vi "UHR-Fleezers Control (host) -Mau_stepping.vi"(0 "Tab Control":T5(tab)) -> ()   [LabVIEW 2013] (continued)
    n1508 = feedback-in #1(w2281) -> ()
    n1509 = local read "AOM X Cal (nm/MHz)"() -> (w2039:dbl)
    n1510 = To Time Stamp(1:w2086) -> (0:w2085:timestamp)
    n1511 = Split 1D Array(array=w2073, index="N El. to Ave.") -> (second subarray=w2076:dbl[])  [unwired: 1 out]
    n1512 = Split 1D Array(array=w2070, index="N El. to Ave.") -> (second subarray=w2075:dbl[])  [unwired: 1 out]
    n1513 = local read "Trap X AI1 (DMA)"() -> (w2074:T13)
    n1514 = Multiply(x=w2148, y="Trap Disp. Downsample") -> (x*y=w2087:dbl)
    "Display Period (s)" <- w2087
    n1515 = Bundle("BD 1 Frequency 1 (MHz)"=w2042, "BD 1 Frequency 2 (MHz)"=w2041) -> (w2043:T45)  [unwired: 1 out]
    n1516 = for "Trap AI" {
      tunnel: [w2695] -> w2275 mode=indexing
      tunnel: w2085 -> [w2685]
      tunnel: "Trap Disp. Downsample" -> [w2693]
      tunnel: w2166 -> [w2691] mode=indexing
      tunnel: w2148 -> [w2690]
      tunnel: w2165 -> [w2689] mode=indexing
      tunnel: w2084 -> [w2688]
      tunnel: [w2687] -> w2123 mode=indexing
      tunnel: w2087 -> [w2686]
      n1517 = Bundle By Name("Y"=w2691, "dt"=w2690) -> (w2692:waveform(dbl))  [unwired: 1 out]
      n1518 = Set Waveform Attribute(5:w2689, 6:w2688, 7:w2692) -> (3:w2687:waveform(dbl))  [unwired: 1 in, 2 out]
      n1519 = call "downsample 1D array - double.vi"("Ave N"=w2693, "Array In"=w2691) -> ("Array Out"=w2694:dbl[])  [unwired: 1 out]
      n1520 = Bundle By Name(cluster=w2687, "t0"=w2685, "Y"=w2694, "dt"=w2686) -> (w2695:waveform(dbl))
    }
    n1521 = call-poly <vilib>:"Mean.vi"("X"=w2075) -> ("mean"=w2063:dbl)  [unwired: 1 out]
    n1522 = call-poly <vilib>:"Mean.vi"("X"=w2076) -> ("mean"=w2064:dbl)  [unwired: 1 out]
    n1523 = Cluster To Array(cluster=w2043) -> (array=w2040:dbl[])
    n1524 = Reciprocal(x=w2087) -> (1/x=→"Trap Disp. Freq. (Hz)":dbl)
    n1525 = local read "Data points/scans (MCL)"() -> (w2253:dbl)
    n1526 = To Fixed-Point(number=w2063) -> (fixed-point=w2061:fxp<+/-,16,1>)  [unwired: 1 in]
    n1527 = To Fixed-Point(number=w2064) -> (fixed-point=w2062:fxp<+/-,16,1>)  [unwired: 1 in]
    n1528 = Bundle("Trap 1 Pos.", "Trap 2 Pos.") -> (w2083:cluster{string, string})  [unwired: 1 out]
    n1529 = Bundle By Name(cluster=w2074, "Set 1"=w2062, "Set 2"=w2061) -> (→"Trap X AI1 (DMA)":T13)
    n1530 = Cluster To Array(cluster=w2083) -> (array=w2080:string[])
    n1531 = for "Trap Position" {
      tunnel: w2089 -> [w2335] mode=indexing
      tunnel: "Trap Disp. Downsample" -> [w2334]
      tunnel: w2087 -> [w2332]
      tunnel: w2085 -> [w2331]
      tunnel: w2084 -> [w2329]
      tunnel: w2080 -> [w2328] mode=indexing
      tunnel: [w2327] -> w2038 mode=indexing
      tunnel: w2040 -> [w2325] mode=indexing
      tunnel: w2039 -> [w2323]
      n1532 = call "downsample 1D array - double.vi"("Ave N"=w2334, "Array In"=w2335) -> ("Array Out"=w2333:dbl[])  [unwired: 1 out]
      n1533 = Subtract(x=w2333, y=w2325) -> (x-y=w2326:dbl[])
      n1534 = Multiply(x=w2323, y=w2326) -> (x*y=w2324:dbl[])
      n1535 = Bundle By Name("Y"=w2324, "dt"=w2332, "t0"=w2331) -> (w2330:waveform(dbl))  [unwired: 1 out]
      n1536 = Set Waveform Attribute(5:w2328, 6:w2329, 7:w2330) -> (3:w2327:waveform(dbl))  [unwired: 1 in, 2 out]
    }
    "Trap Positions" <- w2038
    n1537 = Bundle("APD 1", "APD 2") -> (w2274:cluster{string, string})  [unwired: 1 out]
    n1538 = Cluster To Array(cluster=w2274) -> (array=w2271:string[])
    n1539 = for "APD" {
      tunnel: w2242 -> [w2674] mode=indexing
      tunnel: w2112 -> [w2682]
      tunnel: [w2678] -> w2119 mode=indexing
      tunnel: "APD Disp. Scale" -> [w2679]
      tunnel: w2084 -> [w2677]
      tunnel: w2271 -> [w2676] mode=indexing
      tunnel: "APD Disp. Downsample" -> [w2672]
      tunnel: [w2675] -> w2270
      tunnel: w2085 -> [w2671]
      n1540 = call "integrate 1D array interval - double.vi"("Ave N"=w2672, "Array In"=w2674) -> ("Array Out"=w2673:dbl[])  [unwired: 1 out]
      n1541 = Multiply(x=w2682, y=w2672) -> (x*y=w2675:dbl)
      n1542 = Divide(x=w2673, y=w2679) -> (x/y=w2680:dbl[])
      n1543 = Bundle By Name("t0"=w2671, "Y"=w2680, "dt"=w2675) -> (w2681:waveform(dbl))  [unwired: 1 out]
      n1544 = Set Waveform Attribute(5:w2676, 6:w2677, 7:w2681) -> (3:w2678:waveform(dbl))  [unwired: 1 in, 2 out]
    }
    "APD Display Period (s)" <- w2270
    n1545 = Reciprocal(x=w2270) -> (1/x=→"APD Display Freq. (Hz)":dbl)
    n1546 = local read "Display Period (s)"() -> (w2147:dbl)
    n1547 = Increment(x=w2253) -> (x+1=w2254:dbl)
    n1548 = Index Array(array=w2038, index=0) -> (element=w2036:waveform(dbl))
    n1549 = To Double Precision Float(number=w2163) -> (double precision float=w2162:dbl[])
    n1550 = feedback #2(w2254) -> (w2257:dbl)
    n1551 = Select(t=0, s=w2244, f=w2257) -> (s? t:f=w2250:dbl)
    n1552 = Array Size(array=w2162) -> (size(s)=w2256:i32)
    n1553 = Add(x=w2256, y=w2250) -> (x+y=w2251:dbl)
    n1554 = Unbundle By Name(w2036) -> ("Y"=w2034:dbl[])
    n1555 = feedback #3(w2163) -> (w2240:u32[])
    n1556 = Build Array (concatenate)(w2240, w2163) -> (w2237:u32[])
    n1557 = feedback #4(w2099) -> (w2118:u32[])
    n1558 = Divide(x="Bead Sep. Int. Time (s)", y=w2147) -> (x/y=w2032:dbl)
    n1559 = Build Array (concatenate)(w2118, w2099) -> (w2117:u32[])
    n1560 = Greater?(x=w2251, y=w2253) -> (0:w2252:bool)
    n1561 = feedback #5(w2034) -> (w2035:dbl[])
    n1562 = Build Array (concatenate)(w2034, w2035) -> (w2033:dbl[])
    n1563 = Select(t=w2250, s=w2252, f=w2251) -> (s? t:f=w2249:dbl)
    n1564 = feedback-in #2(w2249) -> ()
    n1565 = Array Size(array=w2237) -> (size(s)=w2234:i32)
    n1566 = Array Size(array=w2163) -> (size(s)=w2236:i32)
    n1567 = local read "MCL Scanning"() -> (w2247:bool)
    n1568 = local read "APD Integration Time (s)"() -> (w2126:dbl)
    n1569 = Build Array (concatenate)(w2119, w2275) -> (w2121:waveform(dbl)[])
    "All Signals" <- w2121
    n1570 = Split 1D Array(array=w2033, index=w2032) -> (first subarray=w2026:dbl[])  [unwired: 1 out]
    n1571 = feedback-in #5(w2026) -> ()
    n1572 = Multiply(x=w2236, y="APD Ave N") -> (x*y=w2235:dbl)
    n1573 = Greater?(x=w2234, y=w2235) -> (0:w2238:bool)
    n1574 = Not(x=w2252) -> (.not. x?=w2246:bool)
    n1575 = To Double Precision Float(number=w2099) -> (double precision float=w2098:dbl[])
    n1576 = call-poly <vilib>:"Mean.vi"("X"=w2026) -> ("mean"=w2025:dbl)  [unwired: 1 out]
    "Mean T1 Position (nm)" <- w2025
    n1577 = Subtract(x=w2026, y=w2025) -> (x-y=w2031:dbl[])
    n1578 = Square(x=w2031) -> (x^2=w2030:dbl[])
    n1579 = And(x=w2246, y=w2247) -> (x .and. y?=w2248:bool)
    n1580 = call-poly <vilib>:"Mean.vi"("X"=w2030) -> ("mean"=w2029:dbl)  [unwired: 1 out]
    n1581 = case shown="True" w2238 {
      tunnel: w2237 -> [w2455 w2462]
      tunnel: [w2455 w2460] -> w2179
      tunnel: w2235 -> [_ w2457]
      tunnel: w2234 -> [_ w2461]
      tunnel: w2117 -> [w2454 w2459]
      tunnel: [w2454 w2456] -> w2114
      frame False {
      }
      frame True {
        n1582 = Subtract(x=w2461, y=w2457) -> (x-y=w2458:dbl)
        n1583 = Array Subset(array=w2462, index=w2458, length=w2457) -> (w2460:u32[])
        n1584 = Array Subset(array=w2459, index=w2458, length=w2457) -> (w2456:u32[])
      }
    }
    n1585 = feedback-in #3(w2179) -> ()
    n1586 = feedback-in #4(w2114) -> ()
    n1587 = Or(x=w2248, y=w2244) -> (x .or. y?=w2245:bool)
    n1588 = Square Root(x=w2029) -> (sqrt(x)=w2028:dbl)
    n1589 = Equal?(x="Tab Control 6", y=T35."High Res Display") -> (x = y?=w2169:bool)
    n1590 = Multiply(x="APD Disp. Scale", y=w2119) -> (x*y=w2128:waveform(dbl)[])
    n1591 = Multiply(x="APD Disp. Downsample", y=w2126) -> (x*y=w2124:dbl)
    n1592 = Multiply(x=10.0, y=w2028) -> (x*y=→"Trap 1 Position RMS (A)":dbl)
    n1593 = Divide(x=w2128, y=w2124) -> (x/y=w2096:waveform(dbl)[])
    n1594 = Index Array(array=w2096, index=0) -> (element=w2106:waveform(dbl))
    n1595 = case "For computing FFTs for display" shown="True" "Compute FFT" {
      tunnel: w2123 -> [_ w3132]
      frame False {
      }
      frame True {
        n1596 = Build Array("FFT 1 Choice 1", "FFT 1 Choice 2", "FFT 2 Choice 1", "FFT 2 Choice 2") -> (w3125:u16[])
        n1597 = Array Size(array=w3132) -> (size(s)=w3131:i32)
        n1598 = feedback-in #6(w3125) -> ()
        n1599 = feedback #6(u16[] [100, 100, 100, 100]) -> (w3126:u16[])
        n1600 = feedback-in #7("# Spectra to Ave.") -> ()
        n1601 = feedback #7("# Spectra to Ave.") -> (w3123:dbl)
        n1602 = Not Equal?(x="# Spectra to Ave.", y=w3123) -> (x != y?=w3122:bool)
        n1603 = Not Equal?(x=w3125, y=w3126) -> (x != y?=w3124:bool)
        n1604 = feedback #8(1.0) -> (w3109:dbl)
        n1605 = Compound Arithmetic op=OR("Reset FFT", w3124, w3122) -> (w3107:bool)
        n1606 = Select(t=1.0, s=w3107, f=w3109) -> (s? t:f=w3111:dbl)
        n1607 = Greater?(x=w3111, y="# Spectra to Ave.") -> (0:w3130:bool)
        n1608 = Increment(x=w3111) -> (x+1=w3110:dbl)
        n1609 = feedback-in #8(w3110) -> ()
        n1610 = local read "DMA Update Period (s)"() -> (w3105:dbl)
        n1611 = Multiply(x="# Spectra to Ave.", y=w3105) -> (x*y=→"Ave. Time (s)":dbl)
        n1612 = Build Array(cluster{"f0":dbl, "df":dbl, "magnitude":dbl[]} {"f0"=0.0, "df"=0.0, "magnitude"=[]} ("PSD")) -> (w3114:cluster{"f0":dbl, "df":dbl, "magnitude":dbl[]}[])
        n1613 = Build Array(w3114, w3114, w3114, w3114) -> (w3116:T46)
        n1614 = feedback #9(w3116) -> (w3121:T46)
        n1615 = for {
          N: 4 -> [_]
          tunnel: w3125 -> [w3154] mode=indexing
          tunnel: w3132 -> [w3155]
          tunnel: w3131 -> [w3157]
          tunnel: w3107 -> [w3150]
          tunnel: w3130 -> [w3149]
          tunnel: "# Spectra to Ave." -> [w3148]
          tunnel: [w3147] -> w3120 mode=indexing
          tunnel: w3121 -> [w3152] mode=indexing
          tunnel: [w3151] -> w3108 mode=indexing
          tunnel: w3111 -> [w3146]
          n1616 = Less?(x=w3154, y=w3157) -> (x < y?=w3156:bool)
          n1617 = Index Array(array=w3155, index=w3154) -> (element=w3153:waveform(dbl))
          n1618 = case shown="True" w3156 {
            tunnel: w3153 -> [_ w3174]
            tunnel: w3152 -> [w3159 w3172]
            tunnel: [w3159 w3160] -> w3151
            tunnel: w3150 -> [_ w3171]
            tunnel: w3149 -> [_ w3164]
            tunnel: w3148 -> [_ w3163]
            tunnel: [cluster{"f0":dbl, "df":dbl, "magnitude":dbl[]} {"f0"=0.0, "df"=0.0, "magnitude"=[]} ("PSD") w3165] -> w3147
            tunnel: w3146 -> [_ w3162]
            frame False {
            }
            frame True {
              n1619 = call <vilib>:"Std Deviation and Variance.vi"("X"=w3174) -> ("mean"=w3175:dbl)  [unwired: 1 in, 2 out]
              n1620 = Subtract(x=w3174, y=w3175) -> (x-y=w3173:waveform(dbl))
              n1621 = xnode "Spectral Measurements"("Signals"=w3173) -> ("PSD"=w3167:cluster{"f0":dbl, "df":dbl, "magnitude":dbl[]})  [unwired: 1 in, 1 out]
              n1622 = case shown="False" w3171 {
                tunnel: w3172 -> [w3184 _]
                tunnel: [w3180 w3189] -> w3160
                tunnel: w3167 -> [w3183 w3190]
                tunnel: w3164 -> [w3182 _]
                frame False {
                  n1623 = Build Array (concatenate)(w3184, w3183) -> (w3181:cluster{"f0":dbl, "df":dbl, "magnitude":dbl[]}[])
                  n1624 = case shown="True" w3182 {
                    tunnel: w3181 -> [w3185 w3188]
                    tunnel: [w3185 w3186] -> w3180
                    frame False {
                    }
                    frame True {
                      n1625 = Delete From Array(array=w3188, index=0) -> (array with subset deleted=w3186:cluster{"f0":dbl, "df":dbl, "magnitude":dbl[]}[])  [unwired: 1 in, 1 out]
                    }
                  }
                }
                frame True {
                  n1626 = Build Array(w3190) -> (w3189:cluster{"f0":dbl, "df":dbl, "magnitude":dbl[]}[])
                }
              }
              n1627 = for {
                tunnel: w3160 -> [w3179] mode=indexing
                tunnel: [w3178] -> w3170 mode=indexing
                workers-P: _ -> [_]
                n1628 = Unbundle By Name(w3179) -> ("magnitude"=w3178:dbl[])
              }
              n1629 = Transpose 2D Array(2D array=w3170) -> (transposed array=w3169:dbl[][])
              n1630 = for {
                tunnel: w3169 -> [w3177] mode=indexing
                tunnel: [w3176] -> w3168 mode=indexing
                workers-P: _ -> [_]
                n1631 = Add Array Elements(numeric array=w3177) -> (sum=w3176:dbl)
              }
              n1632 = Select(t=w3163, s=w3164, f=w3162) -> (s? t:f=w3161:dbl)
              n1633 = Divide(x=w3168, y=w3161) -> (x/y=w3166:dbl[])
              n1634 = Bundle By Name(cluster=w3167, "magnitude"=w3166) -> (w3165:cluster{"f0":dbl, "df":dbl, "magnitude":dbl[]})
            }
          }
        }
        n1635 = case shown="True" w3107 {
          tunnel: w3108 -> [w3139 w3145]
          tunnel: [w3139 w3140] -> w3106
          frame False {
          }
          frame True {
            n1636 = Array Subset(array=w3145, index (row)=0 ("index"), length (row)=4 ("length"), index (col)=0 ("index"), length (col)=1 ("length")) -> (w3140:T46)
          }
        }
        n1637 = feedback-in #9(w3106) -> ()
        n1638 = Split 1D Array(array=w3120, index=2) -> (first subarray=→"FFT 1":cluster{"f0":dbl, "df":dbl, "magnitude":dbl[]}[], second subarray=→"FFT 2":cluster{"f0":dbl, "df":dbl, "magnitude":dbl[]}[])
      }
    }
    n1639 = Index Array(array=w2096, index=1) -> (element=w2104:waveform(dbl))
    n1640 = case "For displaying the high resolution display (no downsampling)" shown="True" w2169 {
      tunnel: w2123 -> [_ w2355]
      frame False {
      }
      frame True {
        n1641 = Index Array(array=w2355, index="High Res. Display") -> (element=w2356:waveform(dbl))
        n1642 = call <vilib>:"Std Deviation and Variance.vi"("X"=w2356) -> ("mean"=w2363:dbl, "standard deviation"=w2368:dbl)  [unwired: 1 in, 1 out]
        "Mean Intensity" <- w2363
        "Sigma" <- w2368
        n1643 = Subtract(x=w2356, y=w2363) -> (x-y=w2362:waveform(dbl))
        n1644 = Select(t=w2362, s="Subtract mean", f=w2356) -> (s? t:f=→"1 Channel":waveform(dbl))
        n1645 = Divide(x=w2368, y=w2363) -> (x/y=→"Sigma/Mean":dbl)
        n1646 = feedback #10(1) -> (w2357:i32)
        n1647 = Greater Or Equal?(x=w2357, y="Slow mean N ave.") -> (x >= y?=w2370:bool)
        n1648 = Increment(x=w2357) -> (x+1=w2372:i32)
        n1649 = Select(t=1, s=w2370, f=w2372) -> (s? t:f=w2359:i32)
        n1650 = feedback-in #10(w2359) -> ()
        n1651 = feedback #11() -> (w2360:waveform(dbl))  [unwired: 1 out]
        n1652 = case shown="Default" w2357 {
          tunnel: [w2375 w2378] -> w2361
          tunnel: w2360 -> [w2377 _]
          tunnel: w2356 -> [w2376 w2378]
          frame Default {
            n1653 = call-poly <vilib>:"Append Waveforms.vi"("waveform B"=w2376, "waveform A"=w2377) -> ("waveform out"=w2375:waveform(dbl))  [unwired: 1 in, 8 out]
          }
          frame 1 {
          }
        }
        n1654 = feedback-in #11(w2361) -> ()
        n1655 = case shown="True" w2370 {
          tunnel: w2361 -> [_ w2374]
          frame False {
          }
          frame True {
            n1656 = call-poly <vilib>:"Mean.vi"("X"=w2374) -> ("mean"=→"Slow mean":dbl)  [unwired: 1 out]
          }
        }
      }
    }
    n1657 = case "For plotting results of scanning MCL" shown="True" w2245 {
      tunnel: w2244 -> [_ w2495]
      tunnel: w2162 -> [_ w2591]
      tunnel: w2253 -> [_ _]
      tunnel: w2123 -> [_ w2565]
      tunnel: w2098 -> [_ w2496]
      tunnel: w2097 -> [_ w2469]
      frame False {
      }
      frame True {
        w2476 = u32 0 items=["Horizontal", "Vertical", "Central", "1st Diagonal", "2nd Diagonal"] ("Type of Symmetry")
        w2504 = u32 0 items=["Horizontal", "Vertical", "Central", "1st Diagonal", "2nd Diagonal"] ("Type of Symmetry")
        w2507 = u32 0 items=["Horizontal", "Vertical", "Central", "1st Diagonal", "2nd Diagonal"] ("Type of Symmetry")
        w2536 = u32 0 items=["Horizontal", "Vertical", "Central", "1st Diagonal", "2nd Diagonal"] ("Type of Symmetry")
        n1658 = Index Array(array=w2565, index=10) -> (element=w2571:waveform(dbl))
        n1659 = Index Array(array=w2565, index=11) -> (element=w2568:waveform(dbl))
        n1660 = local read "Cycles/step (MCL)"() -> (w2521:u64)
        n1661 = Index Array(array=w2565, index="Channel") -> (element=w2567:waveform(dbl))
        n1662 = Unbundle(w2469) -> ("New Image"=w2468:T3, "New Image"=w2467:T3, "New Image"=w2466:T3, "New Image"=w2465:T3)
        n1663 = Unbundle By Name(w2571) -> ("Y"=w2523:dbl[])
        n1664 = Unbundle By Name(w2568) -> ("Y"=w2525:dbl[])
        n1665 = Unbundle By Name(w2567) -> ("Y"=w2530:dbl[])
        n1666 = call "downsample 1D array - double.vi"("Ave N"=w2521, "Array In"=w2523) -> ("Array Out"=w2522:dbl[])  [unwired: 1 out]
        n1667 = call "downsample 1D array - double.vi"("Ave N"=w2521, "Array In"=w2525) -> ("Array Out"=w2524:dbl[])  [unwired: 1 out]
        n1668 = call "downsample 1D array - double.vi"("Ave N"=w2521, "Array In"=w2530) -> ("Array Out"=w2529:dbl[])  [unwired: 1 out]
        n1669 = feedback #12(w2591) -> (w2592:dbl[])
        n1670 = Build Array (concatenate)(w2592, w2591) -> (w2573:dbl[])
        n1671 = feedback #13(w2496) -> (w2498:dbl[])
        n1672 = Build Array (concatenate)(w2498, w2496) -> (w2497:dbl[])
        n1673 = local read "Scan steps (MCL)"() -> (w2478:u64)
        n1674 = Select(t=w2591, s=w2495, f=w2573) -> (s? t:f=w2577:dbl[])
        n1675 = feedback-in #12(w2577) -> ()
        n1676 = Select(t=w2496, s=w2495, f=w2497) -> (s? t:f=w2479:dbl[])
        n1677 = feedback-in #13(w2479) -> ()
        n1678 = local read "Scan lines (y)"() -> (w2464:u64)
        n1679 = local read "N APD Samp/step"() -> (w2480:dbl)
        n1680 = feedback #14(w2522) -> (w2579:dbl[])
        n1681 = Build Array (concatenate)(w2579, w2522) -> (w2570:dbl[])
        n1682 = feedback #15(w2529) -> (w2589:dbl[])
        n1683 = Build Array (concatenate)(w2589, w2529) -> (w2588:dbl[])
        n1684 = feedback #16(w2524) -> (w2581:dbl[])
        n1685 = Build Array (concatenate)(w2581, w2524) -> (w2582:dbl[])
        n1686 = Select(t=w2522, s=w2495, f=w2570) -> (s? t:f=w2526:dbl[])
        n1687 = feedback-in #14(w2526) -> ()
        n1688 = Select(t=w2529, s=w2495, f=w2588) -> (s? t:f=w2528:dbl[])
        n1689 = feedback-in #15(w2528) -> ()
        n1690 = Select(t=w2524, s=w2495, f=w2582) -> (s? t:f=w2527:dbl[])
        n1691 = feedback-in #16(w2527) -> ()
        n1692 = Multiply(x=w2478, y=u64 2) -> (x*y=w2463:u64)
        n1693 = call "integrate 1D array interval - double.vi"("Ave N"=w2480, "Array In"=w2479) -> ("Array Out"=w2491:dbl[])  [unwired: 1 out]
        n1694 = call "integrate 1D array interval - double.vi"("Ave N"=w2480, "Array In"=w2577) -> ("Array Out"=w2576:dbl[])  [unwired: 1 out]
        n1695 = Array Size(array=w2491) -> (size(s)=w2492:i32)
        n1696 = Array Size(array=w2576) -> (size(s)=w2578:i32)
        n1697 = Multiply(x=w2464, y=w2463) -> (x*y=w2494:u64)
        n1698 = Multiply(x=w2464, y=w2463) -> (x*y=w2586:u64)
        n1699 = call-poly <vilib>:"Mean.vi"("X"=w2526) -> ("mean"=w2510:dbl)  [unwired: 1 out]
        n1700 = Subtract(x=w2494, y=w2492) -> (x-y=w2485:u64)
        n1701 = call-poly <vilib>:"Mean.vi"("X"=w2528) -> ("mean"=w2515:dbl)  [unwired: 1 out]
        n1702 = call-poly <vilib>:"Mean.vi"("X"=w2527) -> ("mean"=w2513:dbl)  [unwired: 1 out]
        n1703 = call-poly <vilib>:"Mean.vi"("X"=w2491) -> ("mean"=w2482:dbl)  [unwired: 1 out]
        n1704 = Subtract(x=w2586, y=w2578) -> (x-y=w2520:u64)
        n1705 = call-poly <vilib>:"Mean.vi"("X"=w2576) -> ("mean"=w2517:dbl)  [unwired: 1 out]
        n1706 = Initialize Array(1.0 ("element"), w2485) -> (w2481:dbl[])
        n1707 = Initialize Array(1.0 ("element"), w2520) -> (w2511:dbl[])
        n1708 = Multiply(x=w2481, y=w2482) -> (x*y=w2483:dbl[])
        n1709 = Multiply(x=w2511, y=w2513) -> (x*y=w2514:dbl[])
        n1710 = Multiply(x=w2511, y=w2515) -> (x*y=w2516:dbl[])
        n1711 = Multiply(x=w2511, y=w2510) -> (x*y=w2512:dbl[])
        n1712 = Multiply(x=w2511, y=w2517) -> (x*y=w2518:dbl[])
        n1713 = Build Array (concatenate)(w2526, w2512) -> (w2580:dbl[])
        n1714 = Build Array (concatenate)(w2528, w2516) -> (w2584:dbl[])
        n1715 = Build Array (concatenate)(w2527, w2514) -> (w2583:dbl[])
        n1716 = Build Array (concatenate)(w2491, w2483) -> (w2493:dbl[])
        n1717 = Build Array (concatenate)(w2576, w2518) -> (w2585:dbl[])
        n1718 = Reshape Array(w2580, w2464, w2463) -> (w2546:dbl[][])
        n1719 = Reshape Array(w2493, w2464, w2463) -> (w2489:dbl[][])
        n1720 = Reshape Array(w2584, w2464, w2463) -> (w2538:dbl[][])
        n1721 = Reshape Array(w2583, w2464, w2463) -> (w2553:dbl[][])
        n1722 = Reshape Array(w2585, w2464, w2463) -> (w2563:dbl[][])
        n1723 = Array Subset(array=w2553, index (col)=0 ("index"), length (col)=w2478) -> (w2558:dbl[][])  [unwired: 2 in]
        n1724 = Array Subset(array=w2553, index (col)=w2478) -> (w2556:dbl[][])  [unwired: 3 in]
        n1725 = Array Subset(array=w2538, index (col)=0 ("index"), length (col)=w2478) -> (w2544:dbl[][])  [unwired: 2 in]
        n1726 = Array Subset(array=w2538, index (col)=w2478) -> (w2542:dbl[][])  [unwired: 3 in]
        n1727 = Array Subset(array=w2489, index (col)=0 ("index"), length (col)=w2478) -> (w2488:dbl[][])  [unwired: 2 in]
        n1728 = Array Subset(array=w2489, index (col)=w2478) -> (w2486:dbl[][])  [unwired: 3 in]
        n1729 = Array Subset(array=w2563, index (col)=0 ("index"), length (col)=w2478) -> (w2562:dbl[][])  [unwired: 2 in]
        n1730 = Array Subset(array=w2563, index (col)=w2478) -> (w2560:dbl[][])  [unwired: 3 in]
        n1731 = Array Subset(array=w2546, index (col)=0 ("index"), length (col)=w2478) -> (w2551:dbl[][])  [unwired: 2 in]
        n1732 = Array Subset(array=w2546, index (col)=w2478) -> (w2549:dbl[][])  [unwired: 3 in]
        n1733 = for {
          tunnel: w2558 -> [w2600] mode=indexing
          tunnel: [w2599] -> w2557 mode=indexing
          workers-P: _ -> [_]
          n1734 = Reverse 1D Array(array=w2600) -> (reversed array=w2599:dbl[])
        }
        n1735 = for {
          tunnel: w2544 -> [w2596] mode=indexing
          tunnel: [w2595] -> w2543 mode=indexing
          workers-P: _ -> [_]
          n1736 = Reverse 1D Array(array=w2596) -> (reversed array=w2595:dbl[])
        }
        n1737 = for {
          tunnel: w2488 -> [w2594] mode=indexing
          tunnel: [w2593] -> w2487 mode=indexing
          workers-P: _ -> [_]
          n1738 = Reverse 1D Array(array=w2594) -> (reversed array=w2593:dbl[])
        }
        n1739 = for {
          tunnel: w2562 -> [w2602] mode=indexing
          tunnel: [w2601] -> w2561 mode=indexing
          workers-P: _ -> [_]
          n1740 = Reverse 1D Array(array=w2602) -> (reversed array=w2601:dbl[])
        }
        n1741 = for {
          tunnel: w2551 -> [w2598] mode=indexing
          tunnel: [w2597] -> w2550 mode=indexing
          workers-P: _ -> [_]
          n1742 = Reverse 1D Array(array=w2598) -> (reversed array=w2597:dbl[])
        }
        n1743 = Index Array(array=w2563, index (row)=0) -> (element=→"Waveform Graph":dbl[])  [unwired: 1 in]
        n1744 = Add(x=w2557, y=w2556) -> (x+y=w2555:dbl[][])
        n1745 = Add(x=w2543, y=w2542) -> (x+y=w2541:dbl[][])
        n1746 = Add(x=w2487, y=w2486) -> (x+y=w2471:dbl[][])
        n1747 = Add(x=w2561, y=w2560) -> (x+y=w2535:dbl[][])
        n1748 = Add(x=w2550, y=w2549) -> (x+y=w2548:dbl[][])
        n1749 = Divide(x=w2541, y=2) -> (x/y=w2539:dbl[][])
        n1750 = Divide(x=w2555, y=2) -> (x/y=w2500:dbl[][])
        n1751 = Divide(x=w2548, y=2) -> (x/y=w2502:dbl[][])
        n1752 = To Single Precision Float(number=w2535) -> (single precision float=w2534:sgl[][])
        n1753 = Transpose 2D Array(2D array=w2539) -> (transposed array=→"Data map":dbl[][])
        n1754 = To Single Precision Float(number=w2471) -> (single precision float=w2475:sgl[][])
        n1755 = To Single Precision Float(number=w2500) -> (single precision float=w2506:sgl[][])
        n1756 = To Single Precision Float(number=w2502) -> (single precision float=w2503:sgl[][])
        n1757 = call "IMAQ ArrayToImage"("Image Pixels (Float)"=w2534, "Image"=w2468) -> ("Image Out"=w2537:T3)  [unwired: 8 in, 1 out]
        n1758 = call "IMAQ ArrayToImage"("Image Pixels (Float)"=w2475, "Image"=w2467) -> ("Image Out"=w2477:T3)  [unwired: 8 in, 1 out]
        n1759 = call "IMAQ ArrayToImage"("Image Pixels (Float)"=w2506, "Image"=w2466) -> ("Image Out"=w2508:T3)  [unwired: 8 in, 1 out]
        n1760 = call "IMAQ ArrayToImage"("Image Pixels (Float)"=w2503, "Image"=w2465) -> ("Image Out"=w2505:T3)  [unwired: 8 in, 1 out]
        n1761 = call "IMAQ Symmetry"("Type of Symmetry"=w2536, "Image Src"=w2537) -> ("Image Dst Out"=w2532:T3)  [unwired: 3 in, 1 out]
        n1762 = call "IMAQ Symmetry"("Type of Symmetry"=w2476, "Image Src"=w2477) -> ("Image Dst Out"=w2473:T3)  [unwired: 3 in, 1 out]
        n1763 = call "IMAQ Symmetry"("Type of Symmetry"=w2507, "Image Src"=w2508) -> ("Image Dst Out"=→"Detection Laser X":T3)  [unwired: 3 in, 1 out]
        n1764 = call "IMAQ Symmetry"("Type of Symmetry"=w2504, "Image Src"=w2505) -> ("Image Dst Out"=→"Detection Laser Y":T3)  [unwired: 3 in, 1 out]
        n1765 = call "IMAQ Set Simple Calibration"("Calibration Axis Info"=T36 {"Origin Pixel"={"X"=0.0, "Y"=0.0}, "Angle Relative to Horizontal (deg)"=0.0, "Axis Reference"=0}, "Grid Descriptor"=T37 {"X Step"=0.3, "Y Step"=0.3, "Unit"=enum."Undefined"}, "Image"=w2532) -> ("Calibrated Image"=→"APD 1":T3)  [unwired: 7 in, 1 out]
        n1766 = call "IMAQ Set Simple Calibration"("Calibration Axis Info"=T36 {"Origin Pixel"={"X"=0.0, "Y"=0.0}, "Angle Relative to Horizontal (deg)"=0.0, "Axis Reference"=0}, "Grid Descriptor"=T37 {"X Step"=0.3, "Y Step"=0.3, "Unit"=enum."Undefined"}, "Image"=w2473) -> ("Calibrated Image"=→"APD 2":T3)  [unwired: 7 in, 1 out]
      }
    }
    n1767 = Subtract(x=w2104, y="APD 2 Offset") -> (x-y=w2101:waveform(dbl))
    n1768 = Subtract(x=w2106, y="APD 1 Offset") -> (x-y=w2102:waveform(dbl))
    n1769 = Index Array(array=w2121, index=3) -> (element=w2189:waveform(dbl))
    n1770 = Index Array(array=w2121, index=6) -> (element=w2186:waveform(dbl))
    n1771 = Build Array(w2102, w2101) -> (→"APD Chart":waveform(dbl)[])
    n1772 = Array Size(array=w2179) -> (size(s)=w2233:i32)
    n1773 = call <vilib>:"Std Deviation and Variance.vi"("X"=w2114) -> ("standard deviation"=w2113:dbl)  [unwired: 1 in, 2 out]
    n1774 = Add Array Elements(numeric array=w2114) -> (sum=w2116:u32)
    n1775 = Add Array Elements(numeric array=w2179) -> (sum=w2243:u32)
    n1776 = call <vilib>:"Std Deviation and Variance.vi"("X"=w2179) -> ("standard deviation"=w2178:dbl)  [unwired: 1 in, 2 out]
    n1777 = Divide(x="T1 offset_x (mV)", y=1000.0) -> (x/y=w2190:dbl)
    n1778 = Divide(x=w2113, y=w2112) -> (x/y=w2109:dbl)
    "Rate sigma (Hz) 2" <- w2109
    n1779 = Multiply(x=w2112, y=w2233) -> (x*y=w2115:dbl)
    "Int. Time (s)" <- w2115
    n1780 = Divide(x=w2116, y=w2115) -> (x/y=w2110:dbl)
    "APD 2 Rate (Hz)" <- w2110
    n1781 = Divide(x=w2243, y=w2115) -> (x/y=w2176:dbl)
    "APD 1 Rate (Hz)" <- w2176
    n1782 = Divide(x=w2178, y=w2112) -> (x/y=w2177:dbl)
    "Rate sigma (Hz)" <- w2177
    n1783 = Divide(x=w2109, y=w2110) -> (x/y=→"Sigma/Mean 2":dbl)
    n1784 = Divide(x=w2177, y=w2176) -> (x/y=→"Sigma/Mean":dbl)
    n1785 = Divide(x="T2 offset_x (mV)", y=1000.0) -> (x/y=w2188:dbl)
    n1786 = case shown="1" "Calibration" {
      tunnel: "T1 alpha_x (nm/V)" -> [_ w2431 w2452]
      tunnel: "T1 kappa_x (pN/nm)" -> [_ _ w2442]
      tunnel: "T2 alpha_x (nm/V)" -> [_ w2430 w2450]
      tunnel: "T2 kappa_x (pN/nm)" -> [_ _ w2443]
      tunnel: w2189 -> [w2413 w2428 w2448]
      tunnel: w2186 -> [w2412 w2426 w2446]
      tunnel: [w2413 w2425 w2445] -> w2219
      tunnel: [w2412 w2424 w2444] -> w2218
      tunnel: ["T1 X (V)" ("Label.Text") "T1 X (nm)" ("Label.Text") "T1 X (pN)" ("Label.Text")] -> w2207
      tunnel: ["T2 X (V)" ("Label.Text") "T2 X (nm)" ("Label.Text") "T2 X (pN)" ("Label.Text")] -> w2206
      tunnel: ["Position (V)" ("Label.Text") "Position (nm)" ("Label.Text") "Force (pN)" ("Label.Text")] -> w2208
      tunnel: w2188 -> [_ w2416 w2435]
      tunnel: w2190 -> [_ w2419 w2437]
      tunnel: ["Mean (V)" ("Label.Text") "Mean (nm)" ("Label.Text") "Mean (pN)" ("Label.Text")] -> w2203
      tunnel: ["Difference (V)" ("Label.Text") "Difference (nm)" ("Label.Text") "Difference (pN)" ("Label.Text")] -> w2129
      frame 0, Default {
      }
      frame 1 {
        # "position"
        n1787 = Unbundle By Name(w2428) -> ("Y"=w2432:dbl[])
        n1788 = Unbundle By Name(w2426) -> ("Y"=w2417:dbl[])
        n1789 = Subtract(x=w2432, y=w2419) -> (x-y=w2420:dbl[])
        n1790 = Subtract(x=w2417, y=w2416) -> (x-y=w2418:dbl[])
        n1791 = Multiply(x=w2418, y=w2430) -> (x*y=w2427:dbl[])
        n1792 = Multiply(x=w2431, y=w2420) -> (x*y=w2429:dbl[])
        n1793 = Bundle By Name(cluster=w2426, "Y"=w2427) -> (w2424:waveform(dbl))
        n1794 = Bundle By Name(cluster=w2428, "Y"=w2429) -> (w2425:waveform(dbl))
      }
      frame 2 {
        # "force"
        n1795 = Unbundle By Name(w2448) -> ("Y"=w2453:dbl[])
        n1796 = Unbundle By Name(w2446) -> ("Y"=w2451:dbl[])
        n1797 = Subtract(x=w2451, y=w2435) -> (x-y=w2436:dbl[])
        n1798 = Subtract(x=w2453, y=w2437) -> (x-y=w2438:dbl[])
        n1799 = Compound Arithmetic op=MULTIPLY(w2436, w2450, w2443) -> (w2447:dbl[])
        n1800 = Compound Arithmetic op=MULTIPLY(w2442, w2452, w2438) -> (w2449:dbl[])
        n1801 = Bundle By Name(cluster=w2446, "Y"=w2447) -> (w2444:waveform(dbl))
        n1802 = Bundle By Name(cluster=w2448, "Y"=w2449) -> (w2445:waveform(dbl))
      }
    }
    n1803 = feedback-in #17("Calibration") -> ()
    n1804 = feedback #17(u16 1 ("Calibration")) -> (w2210:u16)
    n1805 = local read "Trap 2 Bead Size (nm)"() -> (w2008:dbl)
    n1806 = local read "Trap 1 Bead Size (nm)"() -> (w2007:dbl)
    n1807 = local read "AOM X Cal (nm/MHz)"() -> (w2005:dbl)
    n1808 = local read "Trap Delta (MHz)"() -> (w2004:dbl)
    n1809 = Not Equal?(x=w2210, y="Calibration") -> (x != y?=w2167:bool)
    n1810 = Multiply(x=w2005, y=w2004) -> (x*y=w2009:dbl)
    n1811 = Add(x=w2008, y=w2007) -> (x+y=w2011:dbl)
    n1812 = Unbundle By Name(w2189) -> ("Y"=w2192:dbl[])
    n1813 = Unbundle By Name(w2186) -> ("Y"=w2195:dbl[])
    n1814 = Divide(x=w2011, y=2.0) -> (x/y=w2006:dbl)
    n1815 = Subtract(x=w2192, y=w2190) -> (x-y=w2193:dbl[])
    n1816 = Subtract(x=w2195, y=w2188) -> (x-y=w2194:dbl[])
    n1817 = disable-structure shown="Enabled" {
      disable-tunnel: [-1.0 ("y") 1.0] -> w2196
      frame Disabled {
      }
      frame Enabled {
      }
    }
    n1818 = Multiply(x=w2194, y="T2 alpha_x (nm/V)") -> (x*y=w2185:dbl[])
    n1819 = Multiply(x="T1 alpha_x (nm/V)", y=w2193) -> (x*y=w2184:dbl[])
    n1820 = Multiply(x=w2218, y=w2196) -> (x*y=w2197:waveform(dbl))
    n1821 = case shown="False" "Read Lateness and Rel Phase" {
      tunnel: w2021 -> [w2379 w2401]
      tunnel: w2020 -> [w2380 w2400]
      tunnel: [w2379 w2399] -> w2182
      tunnel: [w2380 w2398] -> w2181
      frame False {
      }
      frame True {
        n1822 = xnode "Read/Write Control"("FPGA VI Reference In"=w2401, "error in"=w2400) -> ("FPGA VI Reference Out"=w2399:T19, "error out"=w2398:errorcluster, "GI Relative phase"=→"GI relative phase":i16, "Relative phase"=→"Relative phase (AI1)":i16, "AI Late Counter"=→"Late Counter (AI1)":u16, "GI Late Counter"=→"GI Late Counter":u16, "MCL Late Counter"=→"MCL Late Counter":u16, "MCL Relative Phase"=→"Relative Phase (MCL)":i16, "APD Acq Relative Phase"=→"APD Acq Relative Phase":i16, "APD 1 Gate Relative Phase"=→"APD 1 Gate Relative Phase":i16, "APD 2 Gate Relative Phase"=→"APD 2 Gate Relative Phase":i16, "APD Acq Late Counter"=→"APD Acq Late Counter":u16, "APD 1 Gate Late Counter"=→"APD 1 Gate Late Counter":u16, "APD 2 Gate Late Counter"=→"APD 2 Gate Late Counter":u16, "Green FB Relative Phase"=→"Relative phase (Green FB)":i16, "GI Relative phase 2"=→"GI relative phase 2":i16, "GI Late Counter 2"=→"GI Late Counter 2":u16, "Trap Pos FIFO Timeout"=→"Trap Pos FIFO Timeout":u16, "Trap AI FIFO Timeout"=→"Trap AI FIFO Timeout":u16)
      }
    }
    n1823 = Subtract(x=w2185, y=w2184) -> (x-y=w2003:dbl[])
    n1824 = call-poly <vilib>:"Mean.vi"("X"=w2003) -> ("mean"=w2010:dbl)  [unwired: 1 out]
    n1825 = Add(x=w2009, y=w2010) -> (x+y=w2013:dbl)
    n1826 = Subtract(x=w2013, y=w2006) -> (x-y=→"Tether Extension (nm, calculated)":dbl)
    n1827 = Unbundle By Name(w2218) -> ("Y"=w2154:dbl[])
    n1828 = Unbundle By Name(w2219) -> ("Y"=w2155:dbl[])
    n1829 = Build Array(w2219, w2197) -> (→"Force":waveform(dbl)[])
    n1830 = Subtract(x=w2003, y="Offset (nm)") -> (x-y=w2152:dbl[])
    n1831 = call-poly <vilib>:"Mean.vi"("X"=w2154) -> ("mean"=w2133:dbl)  [unwired: 1 out]
    "T2 X" <- w2133
    n1832 = Absolute Value(x=w2155) -> (abs(x)=w2156:dbl[])
    n1833 = Absolute Value(x=w2154) -> (abs(x)=w2157:dbl[])
    n1834 = call-poly <vilib>:"Mean.vi"("X"=w2155) -> ("mean"=w2134:dbl)  [unwired: 1 out]
    "T1 X" <- w2134
    n1835 = Add(x=w2156, y=w2157) -> (x+y=w2158:dbl[])
    n1836 = Bundle By Name(cluster=w2189, "Y"=w2152) -> (w2120:waveform(dbl))
    "Bead Separation" <- w2120
    n1837 = Divide(x=w2158, y=2.0) -> (x/y=→"Vec Mean of T1 T2":dbl[])
    n1838 = case shown="True" w2167 {
      tunnel: w2208 -> [_ w2406]
      tunnel: w2207 -> [_ w2405]
      tunnel: w2206 -> [_ w2404]
      tunnel: w2203 -> [_ w2403]
      tunnel: w2129 -> [_ w2402]
      frame False {
      }
      frame True {
        n1839 = property on="Force" class="WFChart (strict)"("YScale.NameLbl.Text"=w2406) -> ()  [unwired: 2 in, 2 out]
        n1840 = property on="T2 X" class="DigNum (strict)"("Caption.Text"=w2404) -> ()  [unwired: 2 in, 2 out]
        n1841 = property on="T1 X" class="DigNum (strict)"("Caption.Text"=w2405) -> ()  [unwired: 2 in, 2 out]
        n1842 = property on="Mean" class="DigNum (strict)"("Caption.Text"=w2403) -> ()  [unwired: 2 in, 2 out]
        n1843 = property on="Difference" class="DigNum (strict)"("Caption.Text"=w2402) -> ()  [unwired: 2 in, 2 out]
      }
    }
    n1844 = local read "Tether"() -> (w2161:bool)
    n1845 = Absolute Value(x=w2134) -> (abs(x)=w2131:dbl)
    n1846 = Absolute Value(x=w2133) -> (abs(x)=w2130:dbl)
    n1847 = Add(x=w2131, y=w2130) -> (x+y=w2205:dbl)
    n1848 = Subtract(x=w2131, y=w2130) -> (x-y=→"Difference":dbl)
    n1849 = feedback #18(w2152) -> (w2151:dbl[])
    n1850 = Divide(x=w2205, y=2.0) -> (x/y=w2160:dbl)
    "Mean" <- w2160
    n1851 = case shown="True" w2161 {
      tunnel: w2160 -> [_ w2338]
      frame False {
      }
      frame True {
        n1852 = Greater?(x="Lost Tether Alarm Threshold (pN)", y=w2338) -> (0:w2336:bool)
        n1853 = case shown="True" w2336 {
          frame False {
          }
          frame True {
            n1854 = flat-sequence {
              frame #0 {
                # "stop only if saving"
                n1855 = local read "Saving..."() -> (w2351:bool)
                n1856 = And(x=w2351, y="TA Cancel Save?") -> (x .and. y?=w2350:bool)
                n1857 = local write "Stop Saving"(w2350) -> ()
              }
              frame #1 {
                n1858 = case shown="True" "TA Green Off?" {
                  frame False {
                  }
                  frame True {
                    w2354 = FALSE ("Fl. Triggered...")
                    n1859 = local write "Fl. Triggered..."(w2354) -> ()
                    n1860 = property on="Green Laser ON/Interlacing" class="Bool (strict)"("Val(Sgnl)"=w2354) -> ()  [unwired: 2 in, 2 out]
                  }
                }
              }
            }
            n1861 = local read "Time tether formed"() -> (w2345:timestamp)
            n1862 = Get Date/Time In Seconds() -> (seconds since 1Jan1904=w2346:timestamp)
            n1863 = Subtract(x=w2346, y=w2345) -> (x-y=w2344:dbl)
            n1864 = Number To Decimal String(number=w2344) -> (decimal integer string=w2341:string)  [unwired: 1 out]
            n1865 = local read "Messages"() -> (w2348:string)
            n1866 = call <vilib>:"Beep.vi"() -> ()  [unwired: 3 in, 9 out]
            n1867 = Concatenate Strings("Lost tether (" ("Message to add"), w2341, " s)." ("string")) -> (w2343:string)
            n1868 = local write "Tether"(FALSE ("Tether")) -> ()
            n1869 = call "Update messages.vi"("Message to add"=w2343, "Old message string"=w2348) -> ("New message string"=w2347:string)
            n1870 = local write "Messages"(w2347) -> ()
            n1871 = property on="Trap Pos. FB ON" class="Bool (strict)"("Val(Sgnl)"=FALSE ("Value (Signaling)")) -> ()  [unwired: 2 in, 2 out]
          }
        }
      }
    }
    n1872 = Build Array (concatenate)(w2152, w2151) -> (w2150:dbl[])
    n1873 = Split 1D Array(array=w2150, index=w2032) -> (first subarray=w2146:dbl[])  [unwired: 1 out]
    n1874 = feedback-in #18(w2146) -> ()
    n1875 = call-poly <vilib>:"Mean.vi"("X"=w2146) -> ("mean"=w2145:dbl)  [unwired: 1 out]
    "Bead Mean (nm)" <- w2145
    n1876 = Subtract(x=w2146, y=w2145) -> (x-y=w2144:dbl[])
    n1877 = Square(x=w2144) -> (x^2=w2143:dbl[])
    n1878 = call-poly <vilib>:"Mean.vi"("X"=w2143) -> ("mean"=w2142:dbl)  [unwired: 1 out]
    n1879 = Square Root(x=w2142) -> (sqrt(x)=w2141:dbl)
    n1880 = Multiply(x=10.0, y=w2141) -> (x*y=→"RMS (Ang)":dbl)
    n1881 = xnode "Read/Write Control"("FPGA VI Reference In"=w2182, "error in"=w2181) -> ("FPGA VI Reference Out"=w2299:T19, "error out"=w2293:errorcluster, "AI4 Y Sum Set 1"=w2289:i16, "AI4 Y Sum Set 2"=w2288:i16, "AI1 X Set 1"=w2066:fxp<+/-,16,1>, "AI1 X Set 2"=w2065:fxp<+/-,16,1>, "Trap Pos FB Int Signal"=→"Trap Pos FB Int Signal":fxp<+/-,24,9>, "Trap Pos FB Int-Norm Signal"=→"Trap Pos FB Int-Norm Signal":fxp<+/-,16,1>, "Trap Pos FB Action"=w2059:i64, "Scanning"=→"AOD Scanning":bool, "Scan I"=→"AOD Scan I":u64, "Scanning MCL"=w2291:bool, "Scan I (MCL)"=→"MCL Scan I":u64, "Green FB Signals"=w2228:T47)  [unwired: 1 out]
    "MCL Scanning" <- w2291
    "Trap Pos FB Action" <- w2059
    n1882 = local read "AI2 (V)"() -> (w2290:cluster{"Set 1":dbl, "Set 2":dbl})
    n1883 = Bundle By Name(cluster=w2290, "Set 1"=w2289, "Set 2"=w2288) -> (w2286:cluster{"Set 1":dbl, "Set 2":dbl})
    n1884 = Divide(x=w2059, y=327.67) -> (x/y=→"Action (%)":dbl)
    n1885 = local read "Trap X (AI1)"() -> (w2079:T1)
    n1886 = Divide(x=w2286, y=3276.7) -> (x/y=w2285:cluster{"Set 1":dbl, "Set 2":dbl})
    n1887 = local write "AI2 (V)"(w2285) -> ()
    n1888 = Bundle(cluster=w2079, "Trap 1"=w2066, "Trap 2"=w2065) -> (→"Trap X (AI1)":T1)
    n1889 = Divide(x=w2228, y=3276.7) -> (x/y=w2224:T48)
    n1890 = Unbundle By Name(w2224) -> ("Green FB Ch 0"=w2227:dbl, "Green FB Ch 1"=w2226:dbl, "Green FB Ch 2"=w2225:dbl)
    n1891 = Divide(x=w2227, y=w2225) -> (x/y=w2223:dbl)
    n1892 = Divide(x=w2226, y=w2225) -> (x/y=w2222:dbl)
    n1893 = flat-sequence "To save data" {
      tunnel: [w3228] -> w2310
      tunnel: [w3229] -> w2309
      tunnel: w2259 -> [w3222]
      tunnel: w2148 -> [w3226]
      tunnel: ["Save Calibration"] -> w2282
      tunnel: w2279 -> [w3225]
      tunnel: [w3218] -> w2278
      tunnel: [w3215] -> w2277
      tunnel: [w3212] -> w2276
      tunnel: w2258 -> [w3214]
      tunnel: w2165 -> [w3208]
      tunnel: [w3208] -> w2164
      tunnel: ["Start Saving"] -> w2122
      tunnel: [w3202] -> w2048
      tunnel: [w3201] -> w2047
      tunnel: w2310 -> [w3463]
      tunnel: w2309 -> [w3462]
      tunnel: w2049 -> [w3461]
      tunnel: w2282 -> [w3460]
      tunnel: w2278 -> [w3458]
      tunnel: w2277 -> [w3457]
      tunnel: w2276 -> [w3456]
      tunnel: w2135 -> [w3455]
      tunnel: w2174 -> [w3454]
      tunnel: w2164 -> [w3453]
      tunnel: w2122 -> [w3452]
      tunnel: w2120 -> [w3451]
      tunnel: w2096 -> [w3450]
      tunnel: w2048 -> [w3449]
      tunnel: w2047 -> [w3448]
      tunnel: w2046 -> [w3447]
      frame #0 {
        n1894 = Or(x="Save N Sets", y="Start Saving") -> (x .or. y?=w3209:bool)
        n1895 = To Double Precision Float(number=w3225) -> (double precision float=w3219:dbl)
        n1896 = Build Array(w3209, "Save Calibration", w3222, w3214) -> (w3224:bool[])
        n1897 = Compound Arithmetic op=OR("Save Calibration", w3222, w3209, w3214) -> (w3227:bool)
        n1898 = Boolean Array To Number(Boolean array=w3224) -> (number=w3221:u32)
        n1899 = feedback #19(FALSE ("Save APD Data\nwith Trap Data")) -> (w3203:bool)
        n1900 = feedback #20(refnum<k0> refnum) -> (w3230:refnum<file>)
        n1901 = feedback #21(refnum<k0> refnum) -> (w3205:refnum<file>)
        n1902 = feedback #22(FALSE ("Save APD Data\nwith Trap Data")) -> (w3213:bool)
        n1903 = feedback #23(refnum<k0> refnum) -> (w3216:refnum<file>)
        n1904 = feedback #24(0) -> (w3232:i32)
        n1905 = feedback #25() -> (w3220:u32)  [unwired: 1 out]
        n1906 = case shown="True" w3227 {
          tunnel: [w3239 1] -> w3228
          tunnel: w3232 -> [w3241 _]
          tunnel: [w3240 w3259] -> w3229
          tunnel: w3230 -> [w3240 _]
          tunnel: w3226 -> [_ w3279]
          tunnel: w3219 -> [_ w3277]
          tunnel: w3221 -> [_ w3280]
          tunnel: [w3238 w3258] -> w3218
          tunnel: w3220 -> [w3238 _]
          tunnel: [w3237 w3256] -> w3215
          tunnel: w3216 -> [w3237 _]
          tunnel: [w3236 w3255] -> w3212
          tunnel: w3213 -> [w3236 _]
          tunnel: "Start Saving" -> [_ w3253]
          tunnel: w3208 -> [_ w3252]
          tunnel: [w3235 w3243] -> w3201
          tunnel: w3205 -> [w3235 _]
          tunnel: [w3234 w3242] -> w3202
          tunnel: w3203 -> [w3234 _]
          frame False {
            n1907 = Increment(x=w3241) -> (x+1=w3239:i32)
          }
          frame True {
            w3249 = FALSE ("Start Saving")
            w3254 = 9.0  # File Version
            w3262 = FALSE ("prepend array or string size? (T)")
            w3260 = T29."big-endian, network order" ("byte order (0:big-endian, network order)")
            # "write file headers"
            n1908 = local read "BD 1 Frequency 1 (MHz)"() -> (w3276:dbl)
            n1909 = local read "BD 2 Frequency 1 (MHz)"() -> (w3275:dbl)
            n1910 = local read "BD 1 Frequency 2 (MHz)"() -> (w3274:dbl)
            n1911 = local read "BD 2 Frequency 2 (MHz)"() -> (w3273:dbl)
            n1912 = local read "BD 1 Frequency 3 (MHz)"() -> (w3272:dbl)
            n1913 = local read "BD 2 Frequency 3 (MHz)"() -> (w3271:dbl)
            n1914 = Array Size(array=w3252) -> (size(s)=w3251:i32)
            n1915 = To Double Precision Float(number=w3251) -> (double precision float=w3250:dbl)
            n1916 = local write "Save Calibration"(w3249) -> ()
            n1917 = local write "Start Saving"(w3249) -> ()
            n1918 = Build Array("Save APD Data\nwith Trap Data", "Save Trap Pos. Data") -> (w3246:bool[])
            n1919 = Boolean Array To Number(Boolean array=w3246) -> (number=w3245:u32)
            n1920 = Build Array(w3276, w3275, w3274, w3273, w3272, w3271) -> (w3270:dbl[])
            n1921 = case shown="4" w3280 {
              tunnel: w3279 -> [w3351 w3371 w3387 w3425]
              tunnel: w3250 -> [w3356 w3378 w3407 w3444]
              tunnel: w3277 -> [w3355 w3377 w3406 w3443]
              tunnel: [w3352 w3373 w3398 w3435] -> w3268
              tunnel: [w3343 "Cal sets to save" w3388 w3426] -> w3258
              tunnel: w3270 -> [w3353 w3374 w3400 w3437]
              tunnel: "Save APD Data\nwith Trap Data" -> [w3350 _ w3384 w3423]
              tunnel: [w3350 w3365 w3384 w3423] -> w3255
              tunnel: w3254 -> [w3346 w3366 w3382 w3421]
              tunnel: w3253 -> [w3345 _ _ _]
              tunnel: [w3336 w3365 w3381 w3411] -> w3242
              tunnel: "Save Trap Pos. Data" -> [w3336 _ w3381 w3411]
              tunnel: w3245 -> [w3335 _ w3380 w3410]
              frame 1, Default {
                # "timeseries"
                n1922 = case shown="True" "Profile" {
                  tunnel: [w3359 w3362] -> w3340
                  tunnel: [w3359 w3361] -> w3339
                  tunnel: [w3359 w3360] -> w3338
                  tunnel: [w3359 w3364] -> w3337
                  frame False {
                    w3359 = 0.0 ("f")
                  }
                  frame True {
                    n1923 = local read "Current Position"() -> (w3363:dbl[])
                    n1924 = local read "Y change (mm)"() -> (w3364:dbl)
                    n1925 = call "subVI_explode3array.vi"("Array"=w3363) -> ("x"=w3362:dbl, "y"=w3361:dbl, "z"=w3360:dbl)  [unwired: 12 in]
                  }
                }
                n1926 = local read "Save ave N"() -> (w3358:dbl)
                n1927 = Multiply(x=w3358, y=w3351) -> (x*y=w3357:dbl)
                n1928 = To Double Precision Float(number=w3335) -> (double precision float=w3349:dbl)
                n1929 = Build Array(w3346, w3351, w3357, w3356, w3355, 0.0 ("f")) -> (w3354:dbl[])
                n1930 = Build Array(w3349, w3340, w3339, w3338, w3337) -> (w3347:dbl[])
                n1931 = Select(t=u32 4000000000, s=w3345, f="N sets to save") -> (s? t:f=w3343:u32)
                n1932 = Build Array (concatenate)(w3354, w3353, w3347) -> (w3352:dbl[])
              }
              frame 2 {
                w3368 = 0.0 ("f")
                w3365 = FALSE ("Save APD Data\nwith Trap Data")
                # "calibration"
                n1933 = Boolean To (0,1)(Boolean=w3365) -> (0, 1=w3370:i16)
                n1934 = To Double Precision Float(number=w3370) -> (double precision float=w3369:dbl)
                n1935 = Build Array(w3369, w3368, w3368, w3368, w3368) -> (w3367:dbl[])
                n1936 = Build Array(w3366, w3371, w3371, w3378, w3377, 1.0 ("t")) -> (w3375:dbl[])
                n1937 = Build Array (concatenate)(w3375, w3374, w3367) -> (w3373:dbl[])
                "Calibrating Trap..." <- TRUE ("Calibrating...")
              }
              frame 4 {
                w3385 = 0.0 ("f")
                # "write file header for a trap \nraster scan"
                # "scan dir (x/y = 0/1)"
                # "cycles/step"
                # "n scans (f/b)"
                # "steps"
                # "freq. range"
                # "AOD raster scan"
                n1938 = local read "Number of F/B Scans (AOD)"() -> (w3392:u16)
                n1939 = local read "Cycles/step (AOD)"() -> (w3394:u64)
                n1940 = local read "Scan Range (MHz)"() -> (w3397:dbl)
                n1941 = local read "Scan steps (AOD)"() -> (w3396:u64)
                n1942 = local read "Scan BD"() -> (w3404:bool)
                n1943 = local read "Save ave N"() -> (w3409:dbl)
                n1944 = Boolean To (0,1)(Boolean=w3404) -> (0, 1=w3403:i16)
                n1945 = To Double Precision Float(number=w3392) -> (double precision float=w3391:dbl)
                n1946 = To Double Precision Float(number=w3396) -> (double precision float=w3395:dbl)
                n1947 = To Double Precision Float(number=w3394) -> (double precision float=w3393:dbl)
                n1948 = To Double Precision Float(number=w3403) -> (double precision float=w3402:dbl)
                n1949 = Multiply(x=w3409, y=w3387) -> (x*y=w3408:dbl)
                n1950 = To Double Precision Float(number=w3380) -> (double precision float=w3386:dbl)
                n1951 = Build Array(w3386, w3385, w3385, w3385, w3385) -> (w3383:dbl[])
                n1952 = local read "N sets should be saved"() -> (w3389:dbl)
                n1953 = Build Array(w3402, w3397, w3395, w3393, w3391) -> (w3399:dbl[])
                n1954 = Build Array(w3382, w3387, w3408, w3407, w3406, 2.0 ("t")) -> (w3401:dbl[])
                n1955 = Round Toward +Infinity(x=w3389) -> (ceil(x): smallest int >= x=w3390:dbl)
                n1956 = Build Array (concatenate)(w3401, w3400, w3383, w3399) -> (w3398:dbl[])
                n1957 = To Unsigned Long Integer(number=w3390) -> (unsigned 32bit integer=w3388:u32)
              }
              frame 8 {
                w3418 = 0.0 ("f")
                # "MCL raster scan"
                n1958 = local read "Number of scans (MCL)"() -> (w3413:u64)
                n1959 = local read "Scan lines (y)"() -> (w3412:u64)
                n1960 = local read "2D or 1D Scan"() -> (w3415:bool)
                n1961 = local read "Scan Range (V)\n(of steps)"() -> (w3434:dbl)
                n1962 = local read "Fast Scan Dir"() -> (w3441:bool)
                n1963 = local read "Cycles/step (MCL)"() -> (w3431:u64)
                n1964 = local read "Scan steps (MCL)"() -> (w3433:u64)
                n1965 = Select(t=w3412, s=w3415, f=w3413) -> (s? t:f=w3414:u64)
                n1966 = Boolean To (0,1)(Boolean=w3415) -> (0, 1=w3417:i16)
                n1967 = local read "Save ave N"() -> (w3446:dbl)
                n1968 = local read "Initial X"() -> (w3420:dbl)
                n1969 = local read "Initial Y"() -> (w3419:dbl)
                n1970 = To Double Precision Float(number=w3417) -> (double precision float=w3416:dbl)
                n1971 = Boolean To (0,1)(Boolean=w3441) -> (0, 1=w3440:i16)
                n1972 = To Double Precision Float(number=w3414) -> (double precision float=w3429:dbl)
                n1973 = To Double Precision Float(number=w3433) -> (double precision float=w3432:dbl)
                n1974 = To Double Precision Float(number=w3431) -> (double precision float=w3430:dbl)
                n1975 = To Double Precision Float(number=w3440) -> (double precision float=w3439:dbl)
                n1976 = Multiply(x=w3446, y=w3425) -> (x*y=w3445:dbl)
                n1977 = To Double Precision Float(number=w3410) -> (double precision float=w3424:dbl)
                n1978 = local read "N sets should be saved (MCL)"() -> (w3427:dbl)
                n1979 = Build Array(w3424, w3416, w3418, w3418, w3418) -> (w3422:dbl[])
                n1980 = Build Array(w3439, w3434, w3432, w3430, w3429, w3420, w3419) -> (w3436:dbl[])
                n1981 = Build Array(w3421, w3425, w3445, w3444, w3443, 3.0 ("t")) -> (w3438:dbl[])
                n1982 = Round Toward +Infinity(x=w3427) -> (ceil(x): smallest int >= x=w3428:dbl)
                n1983 = Build Array (concatenate)(w3438, w3437, w3422, w3436) -> (w3435:dbl[])
                n1984 = To Unsigned Long Integer(number=w3428) -> (unsigned 32bit integer=w3426:u32)
              }
